vi "test Read I64.vi"(8 "error in (no error)":errorcluster, 11 "TestCase in":refnum<class "Buffer Tests.lvclass">) -> (0 "error out":errorcluster, 3 "TestCase out":refnum<class "Buffer Tests.lvclass">)   [LabVIEW 2017, in "Buffer Tests.lvclass"]
uses:
  Buffer Tests.lvclass
  Classes/Buffer/Buffer.lvclass
  C:/Git/DSF/LabVIEW-Memory/Source/Classes/Pointer/Pointer.lvclass
  Classes/Buffer/Read Buffer 0D I64.vi
  <vilib>/addons/_JKI Toolkits/VI Tester/TestCase.llb/TestCase.lvclass
  LabVIEW-Memory/Source/Classes/Pointer/Pointer.lvclass
  C:/Program Files (x86)/National Instruments/LabVIEW 2017/vi.lib/addons/_JKI Toolkits/VI Tester/TestCase.llb/TestCase.lvclass
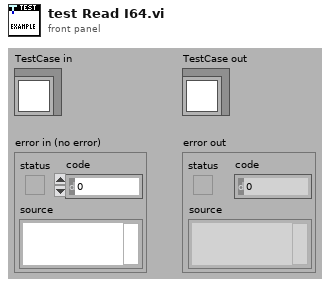
[diagram p1: front panel]
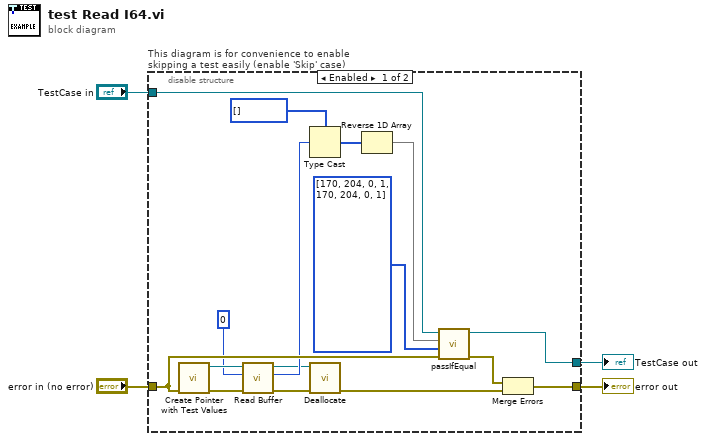
[diagram p0: block diagram]
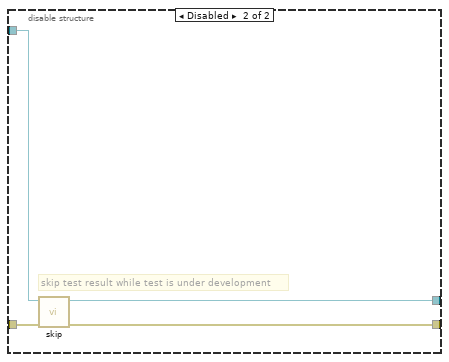
[diagram p2: hidden frame]
diagram:
  n1 = disable-structure "This diagram is for convenience to enable skipping a test easily (enable 'Skip' case)" shown="Enabled" {
    disable-tunnel: "TestCase in" -> [w14 w24]
    disable-tunnel: [w15 w22] -> w2
    disable-tunnel: [w12 w23] -> w3
    disable-tunnel: "error in (no error)" -> [w13 w21]
    frame Enabled {
      n2 = call "Create Pointer with Test Values.vi"("error in (no error)"=w13) -> ("error out"=w9:errorcluster, "Buffer out"=w8:refnum<class "Buffer.lvclass">)  [unwired: 9 in]
      n3 = call-poly "Read Buffer.vi"("error in (no error)"=w9, "dst value in"=i64 0, "Buffer in"=w8) -> ("error out"=w11:errorcluster, "dst value out"=w10:i64, "Buffer out"=w6:refnum<class "Buffer.lvclass">)  [unwired: 5 in, 1 out]
      n4 = Type Cast(type=u8[] [] ("buffer in"), x=w10) -> (*(type *) &x=w20:u8[])
      n5 = call "Deallocate.vi"("error in (no error)"=w11, "Pointer in"=w6) -> ("error out"=w7:errorcluster)  [unwired: 8 in, 1 out]
      n6 = Reverse 1D Array(array=w20) -> (reversed array=w17:u8[])
      n7 = call-dynamic "passIfEqual.vi"("error in (no error)"=w13, "y"=u8[] [170, 204, 0, 1, 170, 204, 0, 1] ("subarray"), "x"=w17, "TestCase in"=w14) -> ("error out"=w16:errorcluster, "TestCase out"=w15:refnum<class "Buffer Tests.lvclass">)  [unwired: 6 in]
      n8 = Merge Errors(w16, w7) -> (w12:errorcluster)
    }
    frame Disabled {
      # "skip test result while test is under development"
      n9 = call <vilib>:"skip.vi"("error in (no error)"=w21, "TestCase in"=w24) -> ("error out"=w23:errorcluster, "TestCase out"=w22:refnum<class "Buffer Tests.lvclass">)  [unwired: 8 in]
    }
  }
  "error out" <- w3
  "TestCase out" <- w2
